vi "Pre-Build Custom Action.vi"(10 "Variant":variant) -> (0 "error out":errorcluster)   [LabVIEW 2024]
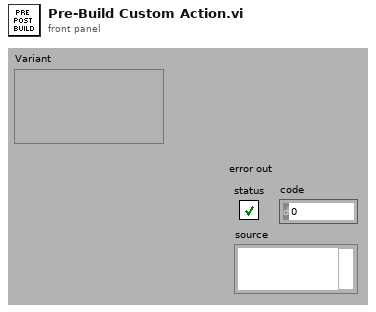
[diagram p1: front panel]
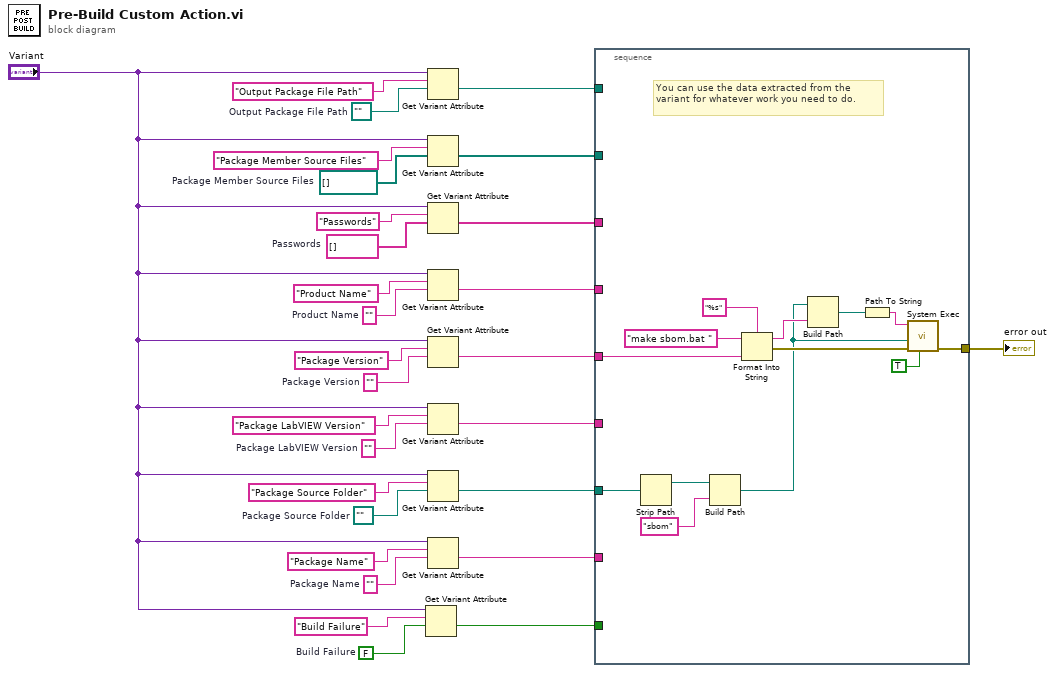
[diagram p0: block diagram]
diagram:
  w4 = FALSE  # Build Failure
  w14 = path ""  # Package Source Folder
  w15 = ""  # Package Name
  w18 = ""  # Package LabVIEW Version
  w20 = ""  # Package Version
  w22 = ""  # Product Name
  w24 = string[] []  # Passwords
  w26 = path[] []  # Package Member Source Files
  w28 = path ""  # Output Package File Path
  n1 = Get Variant Attribute(Variant="Variant", name="Build Failure", default value (empty Variant)=w4) -> (value=w2:bool)  [unwired: 1 in, 3 out]
  n2 = Get Variant Attribute(Variant="Variant", name="Output Package File Path", default value (empty Variant)=w28) -> (value=w13:path)  [unwired: 1 in, 3 out]
  n3 = Get Variant Attribute(Variant="Variant", name="Package Member Source Files", default value (empty Variant)=w26) -> (value=w12:path[])  [unwired: 1 in, 3 out]
  n4 = Get Variant Attribute(Variant="Variant", name="Passwords", default value (empty Variant)=w24) -> (value=w11:string[])  [unwired: 1 in, 3 out]
  n5 = Get Variant Attribute(Variant="Variant", name="Product Name", default value (empty Variant)=w22) -> (value=w10:string)  [unwired: 1 in, 3 out]
  n6 = Get Variant Attribute(Variant="Variant", name="Package Version", default value (empty Variant)=w20) -> (value=w9:string)  [unwired: 1 in, 3 out]
  n7 = Get Variant Attribute(Variant="Variant", name="Package LabVIEW Version", default value (empty Variant)=w18) -> (value=w8:string)  [unwired: 1 in, 3 out]
  n8 = Get Variant Attribute(Variant="Variant", name="Package Source Folder", default value (empty Variant)=w14) -> (value=w7:path)  [unwired: 1 in, 3 out]
  n9 = Get Variant Attribute(Variant="Variant", name="Package Name", default value (empty Variant)=w15) -> (value=w6:string)  [unwired: 1 in, 3 out]
  n10 = stacked-sequence {
    tunnel: w13 -> [_]
    tunnel: w12 -> [_]
    tunnel: w11 -> [_]
    tunnel: w10 -> [_]
    tunnel: w9 -> [w31]
    tunnel: w8 -> [_]
    tunnel: w7 -> [w32]
    tunnel: w6 -> [_]
    tunnel: w2 -> [_]
    tunnel: [w41] -> w1
    frame #0 {
      # "You can use the data extracted from the variant for whatever work you need to do."
      n11 = Strip Path(path=w32) -> (stripped path=w34:path)  [unwired: 1 out]
      n12 = Build Path(base path=w34, name or relative path="sbom") -> (appended path=w30:path)
      n13 = Format Into String(format string="%s", initial string="make sbom.bat ", w31) -> (resulting string=w37:string, error out=w42:errorcluster)  [unwired: 1 in]
      n14 = Build Path(base path=w30, name or relative path=w37) -> (appended path=w36:path)
      n15 = Path To String(path=w36) -> (string=w35:string)
      n16 = call <vilib>:"System Exec.vi"("run minimized? (F)"=TRUE, "error in (no error)"=w42, "working directory"=w30, "command line"=w35) -> ("error out"=w41:errorcluster)  [unwired: 4 in, 3 out]
    }
  }
  "error out" <- w1
